vi "GSP_Wavelength_Global.vi"() -> ()   [LabVIEW 2015]
uses:
  SystemUtil/MotorStates.ctl
  SystemUtil/ThreadStates.ctl
panel:
  in  "WAVMODE REF":refnum<vi>
  in  "WAVMODE":string
  in  "Camera Flex Target":dbl
  in  "Wavelength Thread State":T1
  out "Flexure Active":bool
  in  "Flex_Max":dbl
  in  "B1":dbl
  in  "Grating Min Angle":dbl
  in  "Grating Max Angle":dbl=44.0
  in  "Camera Min Angle":dbl=-1.0
  in  "Camera Max Angle":dbl=88.0
  in  "GS State":T2
  in  "CS State":T2
  in  "GS CPU Temp":dbl
  in  "CS CPU Temp":dbl
  in  "Min Angle difference":dbl=-22.0
  in  "Max Angle difference":dbl=44.0
  in  "Camera Target":dbl
  in  "Grating Target":dbl
  out "WL Online":bool
  in  "Grating Angle":dbl
  in  "GS - Degrees at Home":dbl=20.4 format="%.2f"
  in  "GS - Ticks/Degree":dbl=10000.0 format="%.2f"
  in  "Camera Angle":dbl
  in  "CS - Degrees at Home":dbl=15.0 format="%.2f"
  in  "CS - Ticks per Degree":dbl=28571.43 format="%.2f"
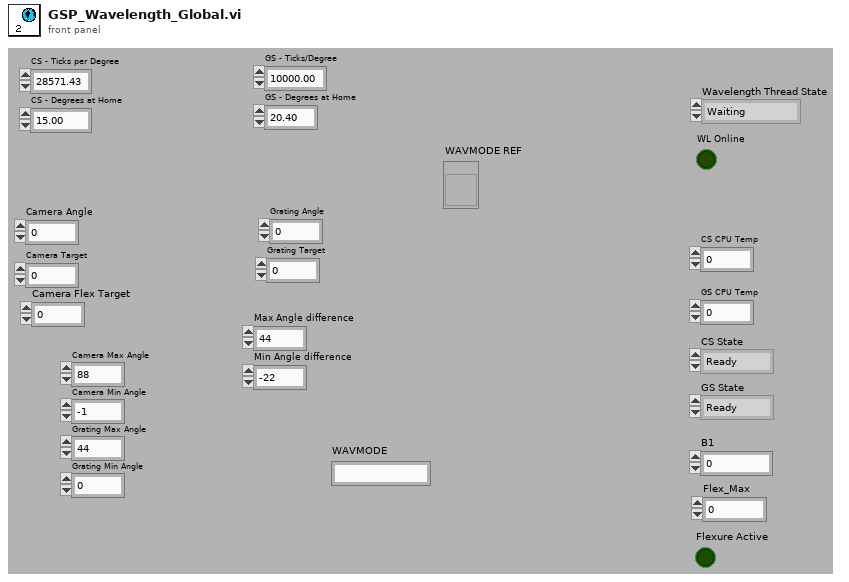
[diagram p1: front panel]
types:
  T1 = typedef "ThreadStates.ctl" = enum16{"Waiting", "Scripting", "Uninitialized", "Error"}
  T2 = typedef "MotorStates.ctl" = enum16{"Ready", "Moving", "Uninitialized", "Error"}
diagram:
